vi "Get Characterization Data.vi"(0 "VISA resource name":refnum<visa-resource-name>, 2 "Enable Temperature Correction?":bool=TRUE, 5 "ACM Path":T3, 7 "S-Parameter":T2, 9 "Characterization Frequencies (for Temp Co)":dbl[](array[numeric]) format="%_6g", 11 "error in (no error)":errorcluster) -> (4 "VISA resource name out":refnum<visa-resource-name>, 8 "S-Par Characterization Data":cdb[](array[numeric]), 15 "error out":errorcluster)   [LabVIEW 2023, in "ACM Visa Driver.lvlib"]
uses:
  ACM Visa Driver.lvlib
  Controls/ACM Paths.ctl
  Controls/ACM S-Parameters.ctl
  HFNetworkAnalysis/Controls/Unit.ctl
  HFNetworkAnalysis/Controls/Quantity.ctl
  HFNetworkAnalysis/Support VIs/Convert Unit (DBL Array).vi
  HFNetworkAnalysis/NI_HFNetworkAnalysis.lvlib
  <vilib>/gmath/NI_Gmath.lvlib
panel:
  in  "Proof for Temp correction/interpolation: The interpolated values (orange) map exactly over the stored temp correction coefficients (blue) and the corrected\ndata (red) swings higher/lower from the original data (white) relative to the value of the correction data. Shown is Path A/Parameter Short.":T1(graph)=[{array[1601 elements], "Characterization Frequencies (for Temp Co)"=array[1601 elements]}, {array[1601 elements], "Characterization Frequencies (for Temp Co)"=array[1601 elements]}, {array[1601 elements], "Characterization Frequencies (for Temp Co)"=array[1601 elements]}, {array[401 elements], "Characterization Frequencies (for Temp Co)"=array[401 elements]}]
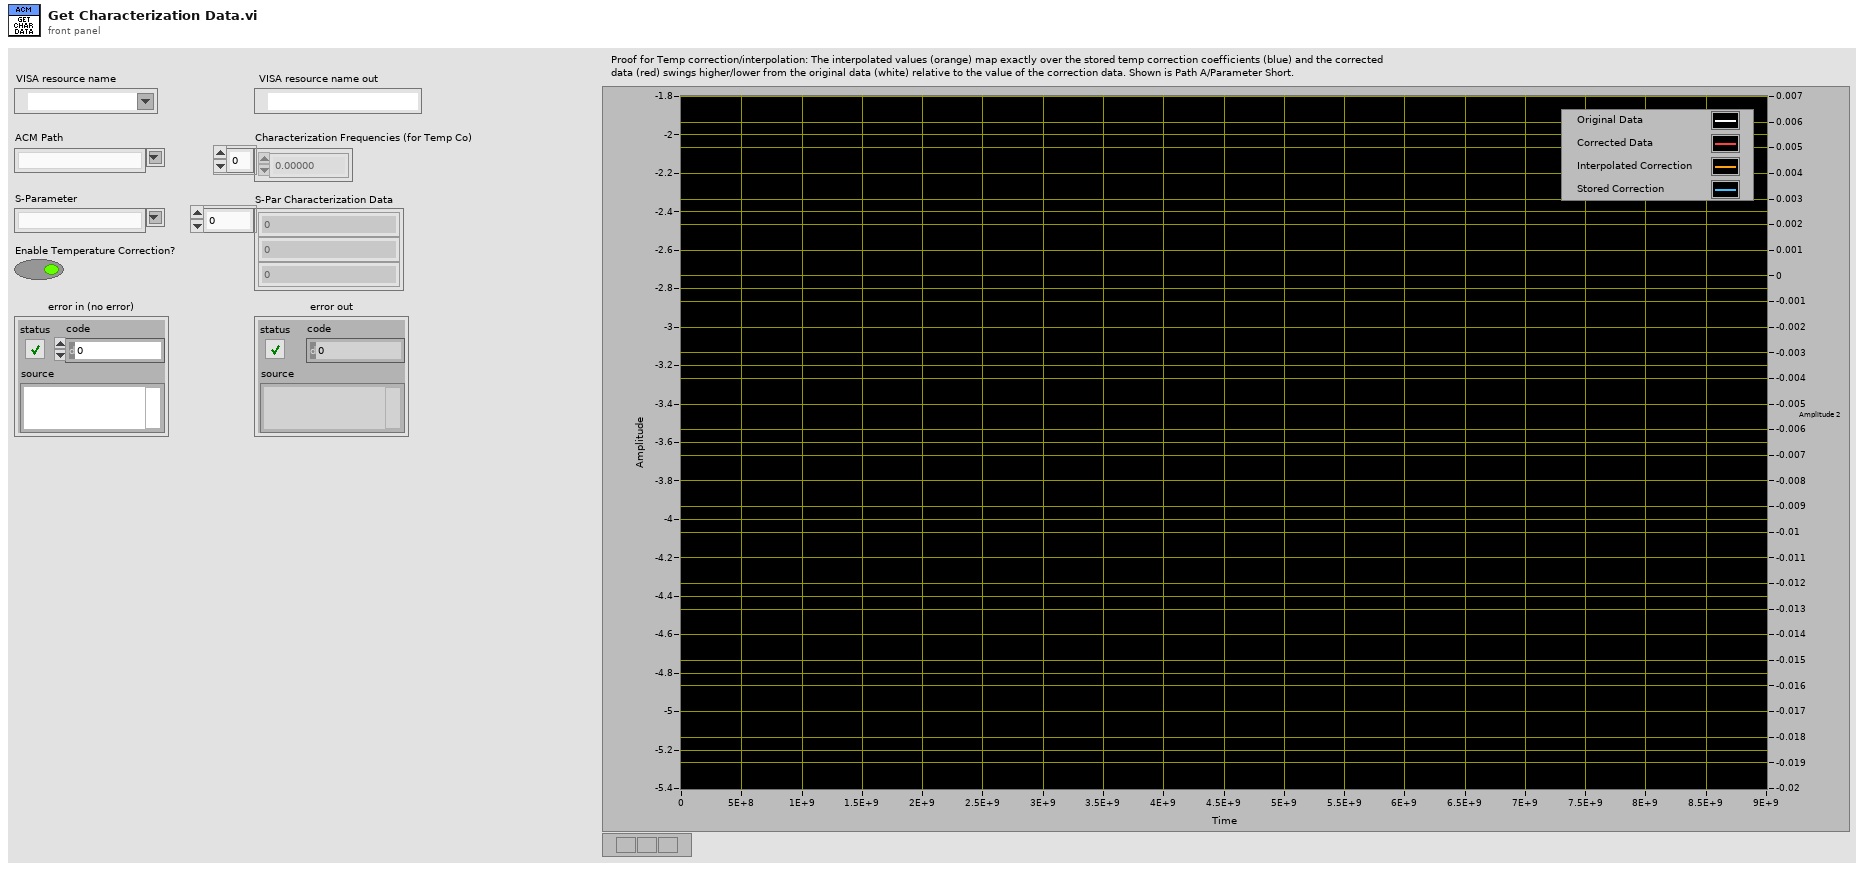
[diagram p1: front panel]
types:
  T1 = cluster{dbl[], "Characterization Frequencies (for Temp Co)":dbl[]}[]
  T2 = typedef "ACM Visa Driver.lvlib/ACM S-Parameters.ctl" = string
  T3 = typedef "ACM Visa Driver.lvlib/ACM Paths.ctl" = string
  T4 = typedef "NI_HFNetworkAnalysis.lvlib/Quantity.ctl" = enum16{"Undefined", "V", "I", "A", "B", "P", "Z", "PowerRatio", "Gamma", "Index"}
  T5 = typedef "NI_HFNetworkAnalysis.lvlib/Unit.ctl" = enum16{"No", "s", "Hz", "V", "A", "Ohm", "W", "dB", "dBV", "dBA", "dBm", "percent", "rad", "deg"}
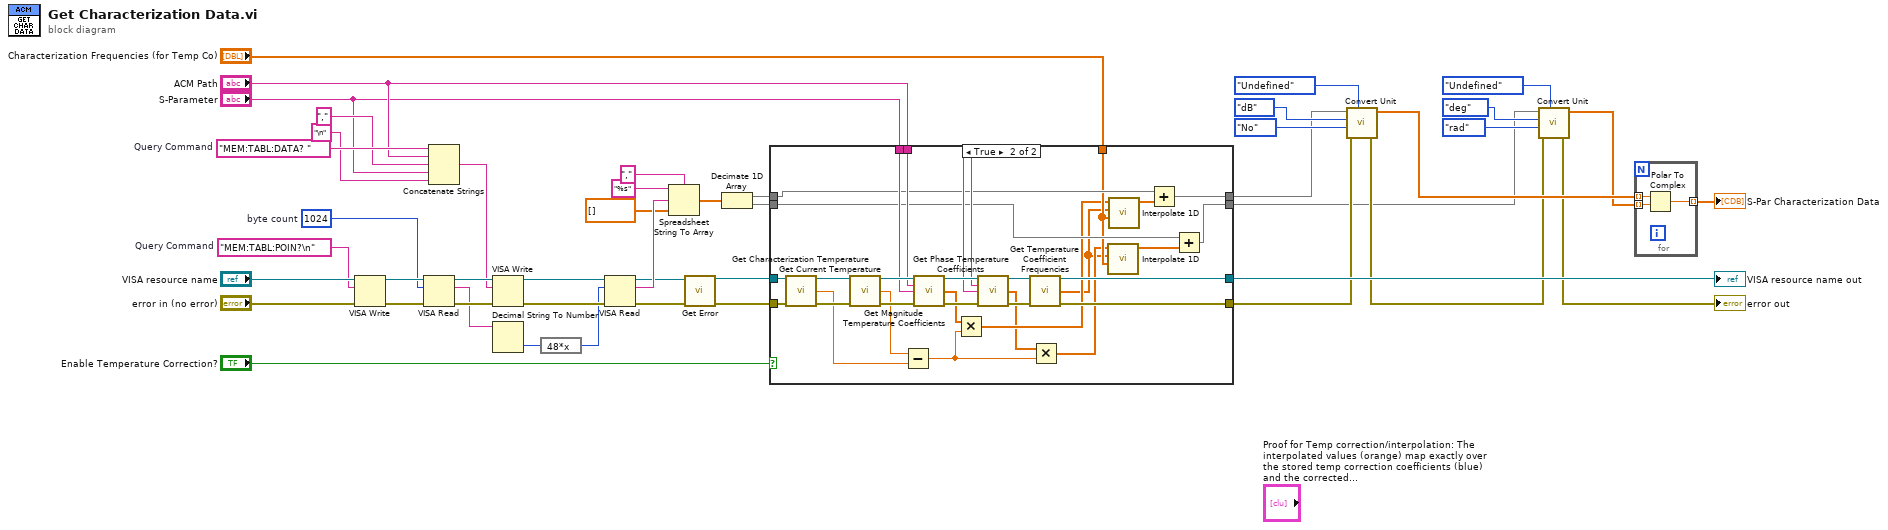
[diagram p0: block diagram]
diagram:
  w37 = "MEM:TABL:DATA? "  # Query Command
  w32 = u32 1024  # byte count
  w41 = "MEM:TABL:POIN?\n"  # Query Command
  n1 = VISA Write(VISA resource name="VISA resource name", write buffer=w41, error in (no error)="error in (no error)") -> (VISA resource name out=w39:refnum<visa-resource-name>, error out=w43:errorcluster)  [unwired: 1 out]
  n2 = VISA Read(VISA resource name=w39, byte count=w32, error in (no error)=w43) -> (VISA resource name out=w38:refnum<visa-resource-name>, read buffer=w33:string, error out=w40:errorcluster)  [unwired: 1 out]
  n3 = Concatenate Strings(w37, "ACM Path", ",", "S-Parameter", "\n") -> (w34:string)
  n4 = VISA Write(VISA resource name=w38, write buffer=w34, error in (no error)=w40) -> (VISA resource name out=w44:refnum<visa-resource-name>, error out=w46:errorcluster)  [unwired: 1 out]
  n5 = Decimal String To Number(string=w33) -> (number=w31:i32)  [unwired: 2 in, 1 out]
  n6 = expression code="48*x"(w31) -> (w30:i32)
  n7 = VISA Read(VISA resource name=w44, byte count=w30, error in (no error)=w46) -> (VISA resource name out=w23:refnum<visa-resource-name>, read buffer=w29:string, error out=w45:errorcluster)  [unwired: 1 out]
  n8 = Spreadsheet String To Array(delimiter (Tab)=",", format string="%s", spreadsheet string=w29, array type (2D Dbl)=dbl[] []) -> (array=w26:dbl[])
  n9 = call "Get Error.vi"("VISA resource name"=w23, "error in (no error)"=w45) -> ("VISA resource name out"=w13:refnum<visa-resource-name>, "error out"=w14:errorcluster)  [unwired: 12 in]
  n10 = Decimate 1D Array(w26) -> (w5:dbl[], w4:dbl[])
  n11 = case shown="True" "Enable Temperature Correction?" {
    tunnel: w14 -> [w50 w80]
    tunnel: w13 -> [w49 w78]
    tunnel: [w49 w62] -> w12
    tunnel: "ACM Path" -> [_ w72]
    tunnel: "S-Parameter" -> [_ w71]
    tunnel: [w50 w61] -> w9
    tunnel: [w51 w66] -> w3
    tunnel: w5 -> [w51 w65]
    tunnel: w4 -> [w48 w59]
    tunnel: [w48 w64] -> w2
    tunnel: "Characterization Frequencies (for Temp Co)" -> [_ w58]
    frame False {
    }
    frame True {
      n12 = call "Get Characterization Temperature.vi"("VISA resource name"=w78, "error in (no error)"=w80) -> ("VISA resource name out"=w76:refnum<visa-resource-name>, "Characterization Temperature (C)"=w69:dbl, "error out"=w79:errorcluster)  [unwired: 11 in]
      n13 = call "Get Current Temperature.vi"("VISA resource name"=w76, "error in (no error)"=w79) -> ("VISA resource name out"=w74:refnum<visa-resource-name>, "Current Temperature (C)"=w70:dbl, "error out"=w77:errorcluster)  [unwired: 11 in]
      n14 = Subtract(x=w70, y=w69) -> (x-y=w67:dbl)
      n15 = call "Get Magnitude Temperature Coefficients.vi"("VISA resource name"=w74, "ACM Path"=w72, "S-Parameter"=w71, "error in (no error)"=w77) -> ("VISA resource name out"=w73:refnum<visa-resource-name>, "Magnitude Coefficients"=w68:dbl[], "error out"=w75:errorcluster)  [unwired: 9 in]
      n16 = Multiply(x=w68, y=w67) -> (x*y=w57:dbl[])
      n17 = call "Get Phase Temperature Coefficients.vi"("VISA resource name"=w73, "ACM Path"=w72, "S-Parameter"=w71, "error in (no error)"=w75) -> ("VISA resource name out"=w63:refnum<visa-resource-name>, "Phase Coefficients"=w56:dbl[], "error out"=w60:errorcluster)  [unwired: 9 in]
      n18 = call "Get Temperature Coefficient Frequencies.vi"("VISA resource name"=w63, "error in (no error)"=w60) -> ("VISA resource name out"=w62:refnum<visa-resource-name>, "Temp Coefficient Frequencies"=w54:dbl[], "error out"=w61:errorcluster)  [unwired: 11 in]
      n19 = Multiply(x=w56, y=w67) -> (x*y=w55:dbl[])
      n20 = call <vilib>:"Interpolate 1D.vi"("xi"=w58, "X"=w54, "Y"=w55) -> ("yi"=w52:dbl[])  [unwired: 6 in, 2 out]
      n21 = call <vilib>:"Interpolate 1D.vi"("xi"=w58, "X"=w54, "Y"=w57) -> ("yi"=w53:dbl[])  [unwired: 6 in, 2 out]
      n22 = Add(x=w65, y=w53) -> (x+y=w66:dbl[])
      n23 = Add(x=w59, y=w52) -> (x+y=w64:dbl[])
    }
  }
  "VISA resource name out" <- w12
  n24 = call-poly "Convert Unit.vi"("Quantity"=Quantity."Undefined", "error in (no error)"=w9, "Target Unit"=Unit."No", "Base Unit"=Unit."dB", "Data"=w3) -> ("error out"=w8:errorcluster, "Converted Data"=w22:dbl[])  [unwired: 2 in]
  n25 = call-poly "Convert Unit.vi"("Quantity"=Quantity."Undefined", "error in (no error)"=w8, "Target Unit"=Unit."rad", "Base Unit"=Unit."deg", "Data"=w2) -> ("error out"=→"error out":errorcluster, "Converted Data"=w15:dbl[])  [unwired: 2 in]
  n26 = for {
    tunnel: w15 -> [w83] mode=indexing
    tunnel: [w82] -> w25 mode=indexing
    tunnel: w22 -> [w81] mode=indexing
    n27 = Polar To Complex(1:w83, 2:w81) -> (0:w82:cdb)
  }
  "S-Par Characterization Data" <- w25
